vi "Test - New Template.vi"(10 "Array":dbl[](array[numeric])) -> (2 "Numeric":dbl)   [LabVIEW 2023]
doc: "This VI is used by the Creating New VI From Template.vi example."
panel:
  # "Select Help>>Show Context Help and move the cursor over  the VI icon to display help for this VI."
  # "This VI serves as a template for the Creating New VI From Template.vi example."
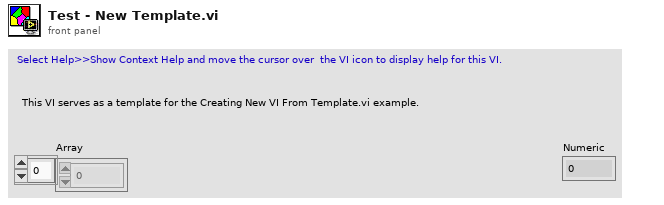
[diagram p1: front panel]
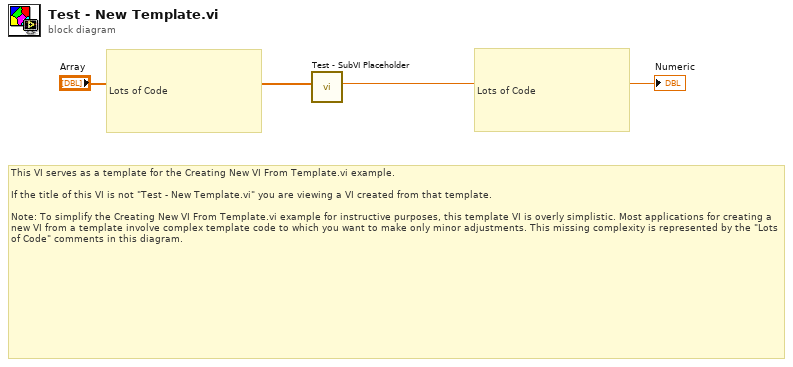
[diagram p0: block diagram]
diagram:
  # "Lots of Code"
  # "This VI serves as a template for the Creating New VI From Template.vi example.\n\nIf the title of this VI is not \"Test - New Template.vi\" you are viewing a VI created from that template.\n\nNote: To simplify the Creating New VI From Template.vi example for instructive purposes, this template VI is overly simplistic. Most applications for creating a new VI from a template involve complex template code to which you want to make only minor adjustments. This missing complexity is represented by the \"Lots of Code\" comments in this diagram."
  # "Lots of Code"
  n1 = call "Test - SubVI Placeholder.vi"("Array"="Array") -> ("Numeric"=→"Numeric":dbl)  [unwired: 10 in]
